vi "rqp_Set Signal Config.vi"(4 "Show in Debugger?":bool=TRUE, 6 "Message Priority":T1=enum."Normal", 7 "Caller in":refnum<class "Worker.lvclass">, 8 "error in":errorcluster, 10 "Data in":T2={"Signal_Config"={"offset"=0.0, "frequency"=10.0, "amplitude"=1.0}, "Signal Type"=enum."Sine Wave"} {"Signal_Config"."amplitude" format="%#_13g"; "Signal_Config"."frequency" format="%#_13g"; "Signal_Config"."offset" format="%0.2p"}, 11 "Analog Signal in":refnum<class "Analog Signal.lvclass">) -> (0 "error out":errorcluster, 3 "dup Analog Signal out":refnum<class "Analog Signal.lvclass">, 5 "dup Caller out":refnum<class "Worker.lvclass">)   [LabVIEW 2023, in "Analog Signal.lvclass"]
doc: "This VI sends a <b>Public API Request</b> message to an MHL case of the Worker that owns this VI.\n---\nSet signal parameter configuration."
uses:
  Analog Signal.lvclass
  C:/Program Files (x86)/National Instruments/LabVIEW 2023/vi.lib/addons/_Workers/Library/Classes/Worker/Worker.lvclass
  <vilib>/addons/_Workers/Library/Classes/Worker/Worker.lvclass
  rqp_Set Signal Config.ctl
  Support/Signal Config.ctl
  Support/Signal Type.ctl
  <vilib>/addons/_Workers/Library/Classes/Message/Priority.ctl
  <vilib>/addons/_Workers/Library/Case Label.ctl
  <vilib>/addons/_Workers/Library/Classes/Message Queue/Message Queue.lvclass
  <vilib>/addons/_Workers/Library/Workers.lvlib
  <vilib>/addons/_Workers/Library/Classes/Message/Message.lvclass
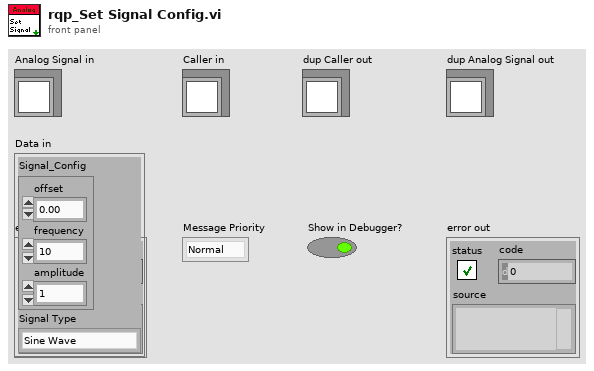
[diagram p1: front panel]
types:
  T1 = typedef "Workers.lvlib/Message.lvclass/Priority.ctl" = enum16{"Low", "Normal", "High"}
  T2 = typedef "Analog Signal.lvclass/rqp_Set Signal Config.ctl" = cluster{"Signal_Config":T3, "Signal Type":T4}
  T3 = typedef "Analog Signal.lvclass/Signal Config.ctl" = cluster{"offset":dbl, "frequency":dbl, "amplitude":dbl}
  T4 = typedef "Analog Signal.lvclass/Signal Type.ctl" = enum16{"Sine Wave", "Square Wave"}
  T5 = typedef "Workers.lvlib/Case Label.ctl" = string
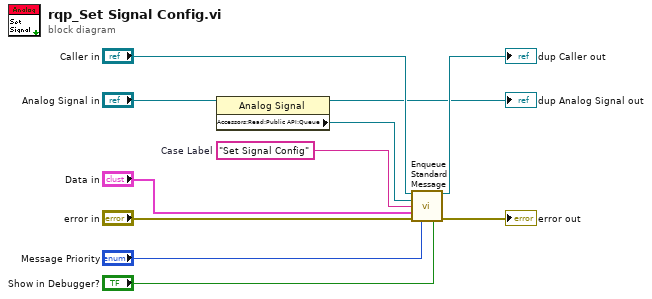
[diagram p0: block diagram]
diagram:
  w1 = T5 "Set Signal Config"  # Case Label
  n1 = property class="Analog Signal"(reference="Analog Signal in") -> (reference out=→"dup Analog Signal out":refnum<class "Analog Signal.lvclass">, "Accessors:Read:Public API:Queue"=w2:refnum<class "Message Queue.lvclass">)  [unwired: 1 in, 1 out]
  n2 = call-dynamic "Enqueue Standard Message.vi"("Worker"="Caller in", "Message Queue"=w2, "Case Label"=w1, "Data"="Data in", "error in (no error)"="error in", "Priority (Normal)"="Message Priority", "Send Message to Debugger? (T)"="Show in Debugger?") -> ("dup Worker out"=→"dup Caller out":refnum<class "Worker.lvclass">, "error out"=→"error out":errorcluster)  [unwired: 7 in]
